vi "Tx.vi"() -> ()   [LabVIEW 2017]
uses:
  <vilib>/addons/Modulation/Digital/Channel Coding/MT Convolutional Encoder (Rate).vi
  <vilib>/addons/Modulation/Analog/support/mod_Set Error Source.vi
  <vilib>/addons/Modulation/Digital/Support/Common/Validators/mod_Validate Bit Stream.vi
  <vilib>/addons/Modulation/Digital/Channel Coding/Convolutional codes/mod_Convolutional encoder.vi
  <vilib>/addons/Modulation/Digital/Channel Coding/Convolutional codes/subVIs/mod_Generate encoder tap connections.vi
  <vilib>/addons/Modulation/Digital/Channel Coding/Convolutional codes/subVIs/mod_Perform convolutional encoding.vi
  <vilib>/addons/Modulation/Digital/Channel Coding/Block codes/subVIs/mod_Buffer block code info (I8).vi
  <vilib>/addons/Modulation/Digital/Channel Coding/Convolutional codes/subVIs/mod_Generate valid reset (convolutional, I8).vi
  <vilib>/addons/Modulation/Digital/General/MT Generate Bits (Fibonacci, PN Order).vi
  <vilib>/addons/Modulation/Digital/Support/Common/Validators/mod_Generate Filter Coefficients Validate.vi
  <vilib>/addons/Modulation/Digital/General/subVIs/mod_Generate Filter Coefficients.vi
  <vilib>/addons/Modulation/Digital/General/MT Generate PSK System Parameters(M).vi
  <vilib>/addons/Modulation/Digital/Channel Coding/Convolutional codes/subVIs/mod_Select known generator matrix.vi
  <vilib>/addons/Modulation/Digital/Support/Common/Validators/mod_Validate Convolutional Encoder prms.vi
  <instrlib>/niUSRP/niUSRP Write Tx Data (CDB Cluster).vi
  <vilib>/addons/Modulation/niDMT.lvlib
panel:
  out "Constellation Graph":T1(graph)
  out "Transmitted Signal":cluster{"t0":dbl, "dt":dbl, "Y":dbl[]}(graph)
  in  "stop":bool
  in  "active antenna":string
  in  "gain":dbl format="%#_6f"
  in  "carrier frequency":dbl=100000.0 format="%#_6p"
  in  "IQ rate":dbl=100000.0 format="%#_6p"
  in  "device names":refnum<k15>
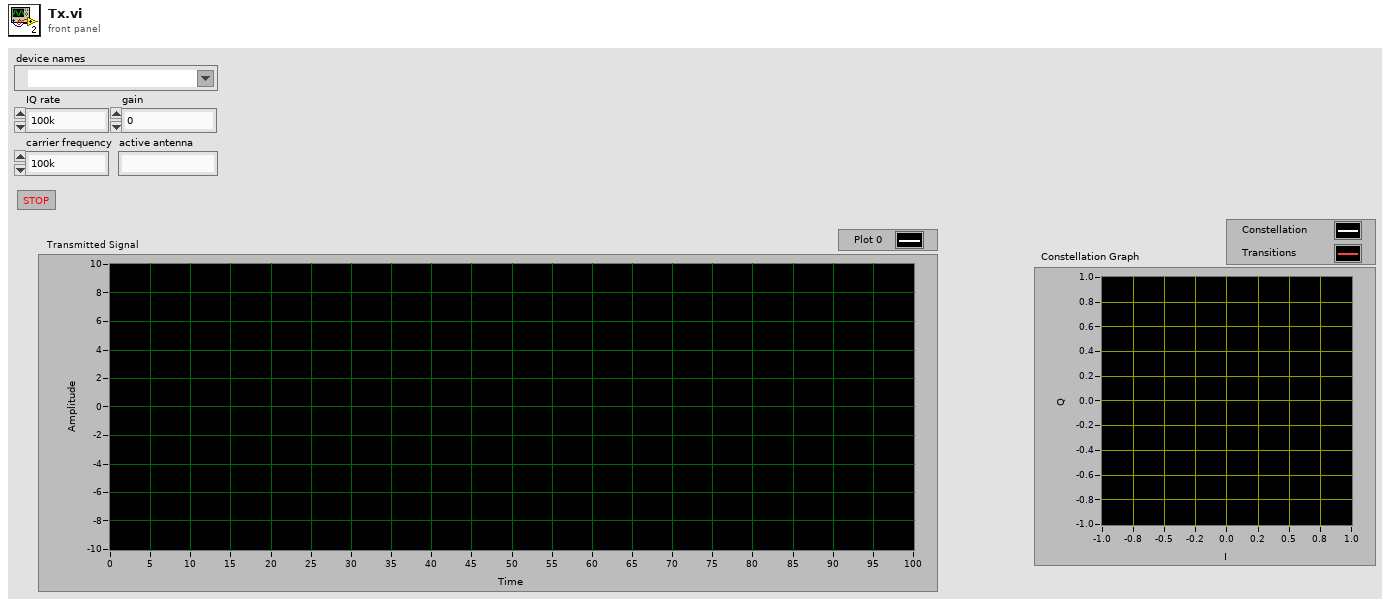
[diagram p1: front panel]
types:
  T1 = cluster{"Decimated Array":dbl[], "Decimated Array":dbl[]}[]
  T2 = enum16{"none", "Raised Cosine", "Root Raised Cos", "Gaussian"}
  T3 = enum16{"FSK", "PSK", "QAM", "MSK", "PAM", "ASK", "CPM"}
  T4 = cluster{"samples per symbol (16)":i32, "symbol map":cdb[], "differential PSK":enum16{"disable", "enable"}, "PSK type":u16}
  T5 = typedef "niAMT.lvlib/Complex Data Waveform.ctl" = cluster{"t0":dbl, "dt":dbl, "Y":cdb[]}
  T6 = cluster{"constellation":dbl[], "oversampled data":dbl[]}[]
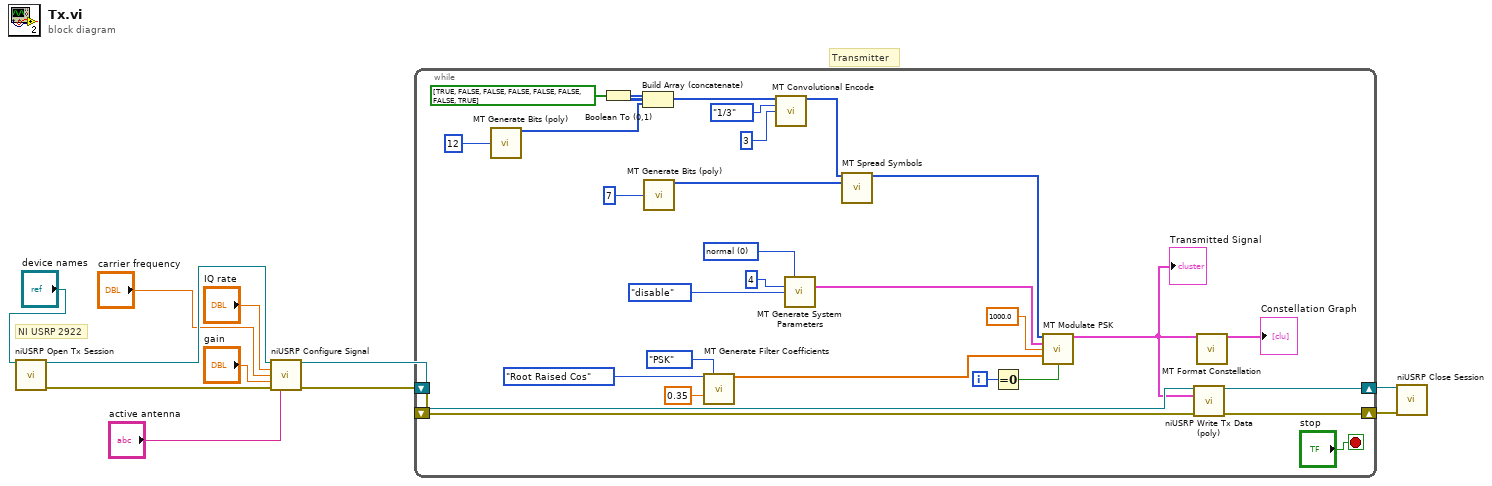
[diagram p0: block diagram]
diagram:
  # "Transmitter"
  # "NI USRP 2922"
  n1 = call <instrlib>:"niUSRP Open Tx Session.vi"("device names"="device names") -> ("session handle out"=w11:refnum<k15>, "error out"=w10:errorcluster)  [unwired: 13 in]
  n2 = call <instrlib>:"niUSRP Configure Signal.vi"("session handle"=w11, "IQ rate"="IQ rate", "carrier frequency"="carrier frequency", "gain"="gain", "error in (no error)"=w10, "active antenna"="active antenna") -> ("session handle out"=w9:refnum<k15>, "error out"=w7:errorcluster)  [unwired: 5 in, 3 out]
  n3 = while {
    shift-right: [w39] -> w8
    shift-left: w9 -> [w40]
    shift-right: [w37] -> w6
    shift-left: w7 -> [w38]
    i -> [w15]
    stop <- "stop" stop-if-true
    w32 = u16 0 items=["normal", "shifted", "offset"] ("PSK type")
    n4 = call-poly <vilib>:"MT Generate Bits (poly).vi"("PN sequence order"=12) -> ("output bit stream"=w16:i8[])  [unwired: 12 in, 2 out]
    n5 = Boolean To (0,1)(Boolean=bool[] [TRUE, FALSE, FALSE, FALSE, FALSE, FALSE, FALSE, TRUE]) -> (0, 1=w22:i16[])
    n6 = Build Array (concatenate) "Build Array"(w22, w16) -> (w20:i16[])
    n7 = call-poly <vilib>:"MT Generate Bits (poly).vi"("PN sequence order"=7) -> ("output bit stream"=w26:i8[])  [unwired: 12 in, 2 out]
    n8 = call <vilib>:"MT Generate Filter Coefficients.vi"("pulse shaping filter (none)"=T2."Root Raised Cos", "modulation type"=T3."PSK", "filter parameter"=0.35) -> ("pulse shaping filter coefficients"=w17:dbl[])  [unwired: 10 in, 2 out]
    n9 = call-poly <vilib>:"MT Convolutional Encode.vi"("input bit stream"=w20, "rate (k/n)"=enum16{"1/2", "1/3", "1/4", "2/3", "3/4"}."1/3", "constraint length (K)"=3) -> ("output bit stream"=w18:i8[])  [unwired: 10 in, 2 out]
    n10 = call-poly <vilib>:"MT Generate System Parameters.vi"("PSK type"=w32, "M-PSK (4)"=4, "differential PSK"=enum16{"disable", "enable"}."disable") -> ("PSK system parameters"=w14:T4)  [unwired: 10 in, 2 out]
    n11 = call <vilib>:"MT Spread Symbols.vi"("input bit stream"=w18, "spreading code"=w26) -> ("output chip stream"=w19:i8[])  [unwired: 12 in, 1 out]
    n12 = Equal To 0?(x=w15) -> (x = 0?=w21:bool)
    n13 = call <vilib>:"MT Modulate PSK.vi"("input bit stream"=w19, "PSK system parameters"=w14, "symbol rate (Hz)"=1000.0, "pulse shaping filter coefficients"=w17, "reset? (T)"=w21) -> ("output complex waveform"=w12:T5)  [unwired: 8 in, 2 out]
    "Transmitted Signal" <- w12
    n14 = call-poly <instrlib>:"niUSRP Write Tx Data (poly).vi"("session handle"=w40, "data"=w12, "error in (no error)"=w38) -> ("session handle out"=w39:refnum<k15>, "error out"=w37:errorcluster)  [unwired: 11 in]
    n15 = call <vilib>:"MT Format Constellation.vi"("waveform"=w12) -> ("constellation graph"=→"Constellation Graph":T6)  [unwired: 13 in, 1 out]
  }
  n16 = call <instrlib>:"niUSRP Close Session.vi"("session handle"=w8, "error in (no error)"=w6) -> ()  [unwired: 13 in, 1 out]
